vi "Read Set IED watchdogReset Msg.vi"(11 "SCADA Sub Abstract in":refnum<class "Device Communication and Control Abstract.lvclass">) -> (2 "Set IED watchdogReset Msg":refnum<class "Set IED watchdogReset Msg.lvclass">, 3 "SCADA Sub Abstract out":refnum<class "Device Communication and Control Abstract.lvclass">)   [LabVIEW 2018, in "Device Communication and Control Abstract Actor.lvlib" / "Device Communication and Control Abstract.lvclass"]
uses:
  Device Communication and Control Abstract.lvclass
  Device Communication and Control Abstract Messages/Set IED watchdogReset Msg/Set IED watchdogReset Msg.lvclass
  Device Communication and Control Abstract.lvclass/Device Communication and Control Abstract.ctl
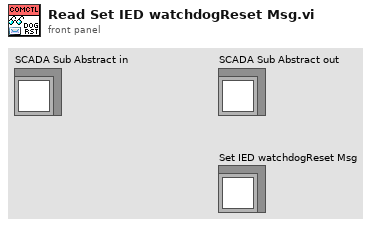
[diagram p1: front panel]
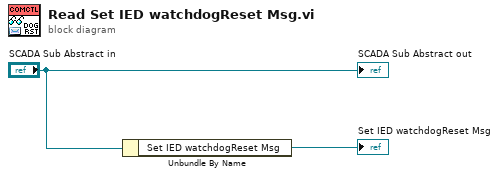
[diagram p0: block diagram]
diagram:
  n1 = Unbundle By Name("SCADA Sub Abstract in") -> ("Set IED watchdogReset Msg"=→"Set IED watchdogReset Msg":refnum<class "Set IED watchdogReset Msg.lvclass">)
  "SCADA Sub Abstract out" <- "SCADA Sub Abstract in"
